vi "Test Person Updates Status on Trigger Broadcast.vi"(8 "error in (no error)":errorcluster, 11 "Worker Test In":refnum<class "Worker Test.lvclass">) -> (0 "error out":errorcluster, 3 "Worker Test Out":refnum<class "Worker Test.lvclass">)   [LabVIEW 2020]
uses:
  Worker Test.lvclass
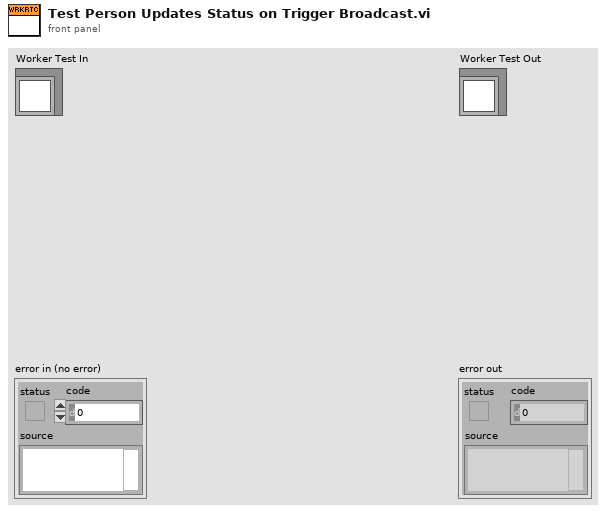
[diagram p1: front panel]
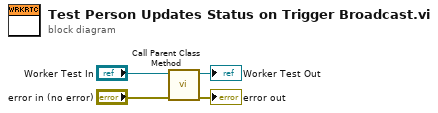
[diagram p0: block diagram]
diagram:
  n1 = call-parent "Call Parent Class Method"("error in (no error)"="error in (no error)", "Person Test In"="Worker Test In") -> ("error out"=→"error out":errorcluster, "Person Test Out"=→"Worker Test Out":refnum<class "Worker Test.lvclass">)  [unwired: 8 in]
